vi "Read Tboard.vi"(8 "error in (no error)":errorcluster, 11 "CR5 Data in":refnum<class "CR5 Data.lvclass">) -> (0 "error out":errorcluster, 2 "Tboard":dbl, 3 "CR5 Data out":refnum<class "CR5 Data.lvclass">)   [LabVIEW 2019, in "CR5 Data.lvclass"]
uses:
  CR5 Data.lvclass
  CR5 Data.lvclass/CR5 Data.ctl
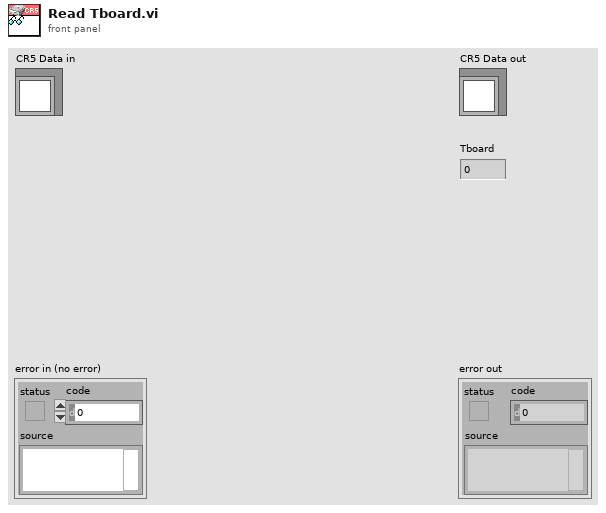
[diagram p1: front panel]
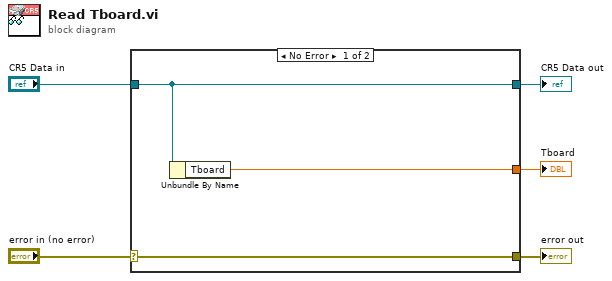
[diagram p0: block diagram]
diagram:
  n1 = case shown="No Error" "error in (no error)" {
    selector: "error in (no error)" -> [w8 w9]
    tunnel: [w8 w9] -> w4
    tunnel: [w7 w10] -> w2
    tunnel: "CR5 Data in" -> [w7 w10]
    tunnel: [w6 _] -> w1
    frame No Error {
      n2 = Unbundle By Name(w7) -> ("Tboard"=w6:dbl)
    }
    frame Error {
    }
  }
  "error out" <- w4
  "CR5 Data out" <- w2
  "Tboard" <- w1
